vi "PalardyGainSchedule.vi"(9 "gainset_negative":cluster{"kp":dbl, "ki":dbl}, 10 "gainset_positive":cluster{"kp":dbl, "ki":dbl}, 11 "error":dbl) -> (3 "chosen_gainset":cluster{"kp":dbl, "ki":dbl})   [LabVIEW 2012]
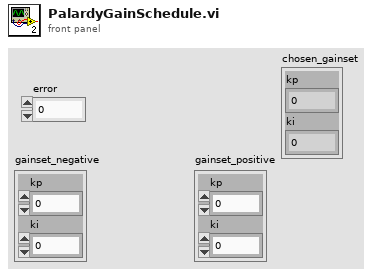
[diagram p1: front panel]
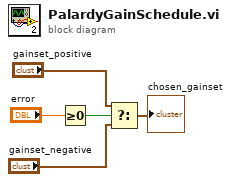
[diagram p0: block diagram]
diagram:
  n1 = Greater Or Equal To 0?(x="error") -> (x >= 0?=w4:bool)
  n2 = Select(t="gainset_positive", s=w4, f="gainset_negative") -> (s? t:f=→"chosen_gainset":cluster{"kp":dbl, "ki":dbl})
